vi "Create_image_legend.vi"(3 "Catégories":string[](array[string])=["Catégorie 1", "Catégorie 2", "Catégorie 3", "Catégorie 4"]) -> (1 "new picture":picture)   [LabVIEW 2024]
uses:
  <vilib>/Math Plots/3D Math Plots/3D Pie/3D Pie XCtrl/3D Pie.xctl
panel:
  out "Nombre de véhicules Total":refnum<class "3D Plot Datatype.lvclass">[](xcontrol)
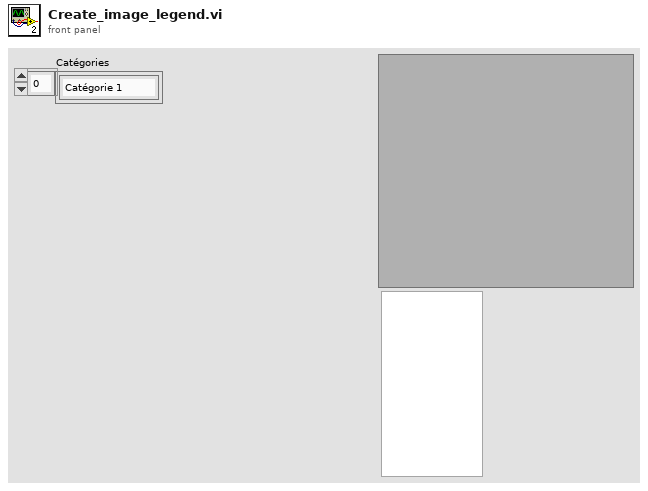
[diagram p1: front panel]
types:
  T1 = cluster{"Immatricule":string, "Color":u32, bool}[]
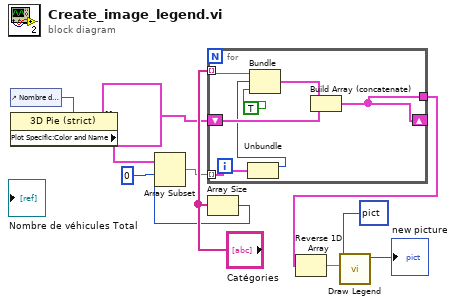
[diagram p0: block diagram]
diagram:
  n1 = control-ref of="Nombre de véhicules Total"() -> (w11:refnum<vi>)
  n2 = property class="3D Pie (strict)"(reference=w11) -> ("Plot Specific:Color and Name"=w5:cluster{"Color":u32, "String":string}[])  [unwired: 1 in, 2 out]
  n3 = Array Size(array="Catégories") -> (size(s)=w7:i32)
  n4 = Array Subset(array=w5, index=0, length=w7) -> (w4:cluster{"Color":u32, "String":string}[])
  n5 = for {
    tunnel: "Catégories" -> [w18] mode=indexing
    shift-right: [w15] -> _
    shift-left: T1 [] -> [w16]
    tunnel: [w15] -> w2
    tunnel: w4 -> [w12] mode=indexing
    n6 = Unbundle(w12) -> ("Color"=w13:u32)  [unwired: 1 out]
    n7 = Bundle("Immatricule"=w18, "Color"=w13, TRUE) -> (w17:cluster{"Immatricule":string, "Color":u32, bool})  [unwired: 1 in]
    n8 = Build Array (concatenate)(w17, w16) -> (w15:T1)
  }
  n9 = Reverse 1D Array(array=w2) -> (reversed array=w1:T1)
  n10 = call <vilib>:"Draw Legend.vi"("plot info"=w1, "picture"=picture data[5B]) -> ("new picture"=→"new picture":picture)  [unwired: 9 in]
